vi "integer_time_to_string.vi"(8 "error in (no error)":errorcluster, 10 "Time (s)":u16) -> (0 "error out":errorcluster, 2 "Time string (mm:ss)":string)   [LabVIEW 2018]
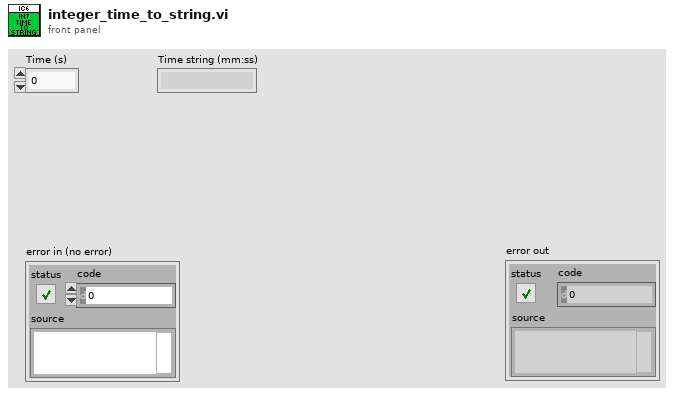
[diagram p1: front panel]
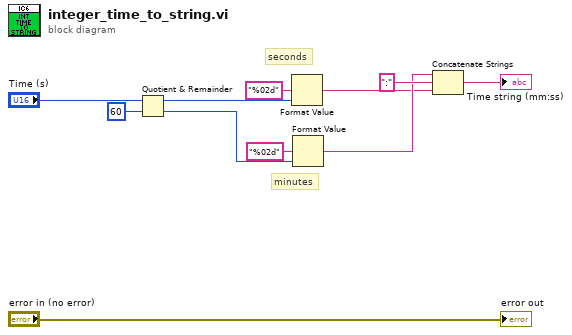
[diagram p0: block diagram]
diagram:
  # "seconds"
  # "minutes"
  n1 = Quotient & Remainder(x="Time (s)", y=u16 60) -> (x-y*floor(x/y)=w3:u16, floor(x/y)=w7:u16)
  n2 = Format Value(format string="%02d", value (0)=w3) -> (output string=w2:string)  [unwired: 1 in]
  n3 = Format Value(format string="%02d", value (0)=w7) -> (output string=w5:string)  [unwired: 1 in]
  n4 = Concatenate Strings(w5, ":" ("string"), w2) -> (→"Time string (mm:ss)":string)
  "error out" <- "error in (no error)"
